vi "CAN_Command Standard.vi"(0 "Write":refnum<k21>, 1 "ID Response":string="18DAF255", 2 "Expression":string, 3 "CAN Command":string, 5 "Read":refnum<k21>, 9 "ID Request":string="18DA55F2", 11 "Numeric Request":u32 format="%x", 12 "Extended":bool=TRUE) -> (4 "Read out":refnum<k21>, 6 "Write out":refnum<k21>, 10 "ID String":string, 13 "Error Out":errorcluster, 14 "Timestamp":timestamp, 15 "Data String":string)   [LabVIEW 2023]
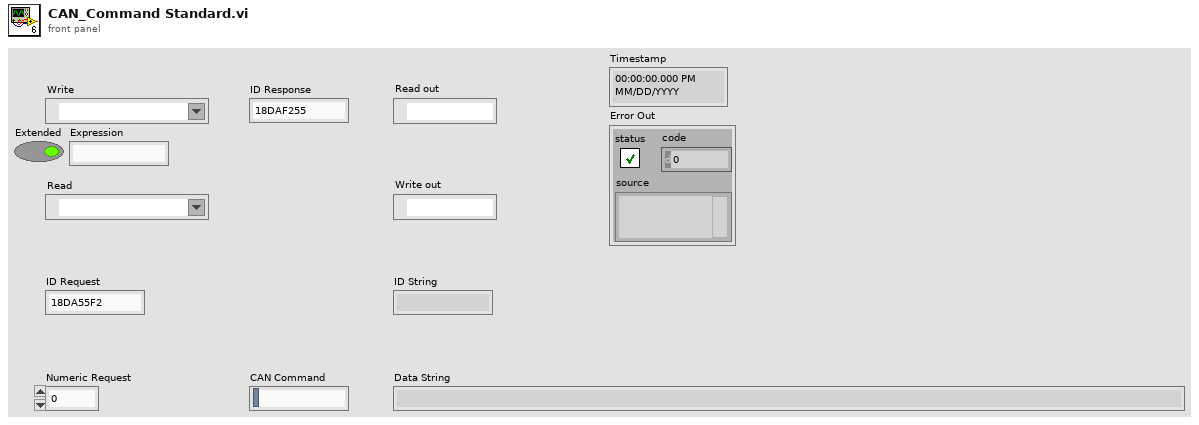
[diagram p1: front panel]
types:
  T1 = typedef "XNET Frame CAN.ctl" = cluster{"timestamp":timestamp, "payload":u8[], "identifier":u32, "type":T2, "extended?":bool, "echo?":bool}
  T2 = typedef "XNET Frame Type CAN.ctl" = u8
  T3 = cluster{"data[0]":T1, "data[1]":T1, "data[2]":T1, "data[3]":T1, "data[4]":T1, "data[5]":T1, "data[6]":T1, "data[7]":T1, "data[8]":T1}
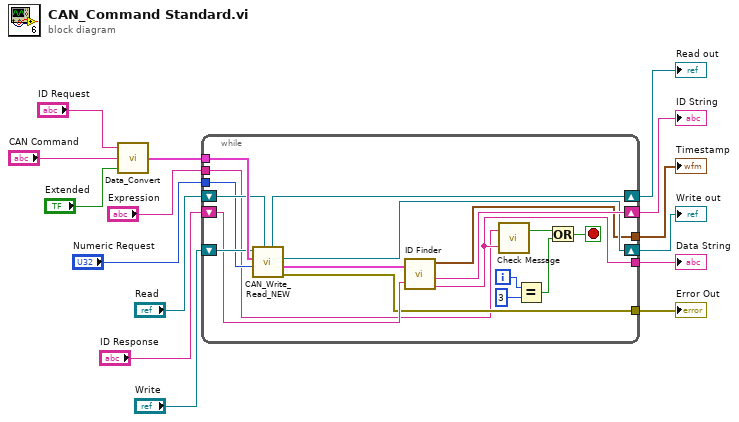
[diagram p0: block diagram]
diagram:
  n1 = call "Data_Convert.vi"("Extended"="Extended", "string"="CAN Command", "ID"="ID Request") -> ("CAN frame"=w13:T1)
  n2 = while {
    tunnel: [w17] -> w14
    tunnel: w13 -> [w31]
    tunnel: "Numeric Request" -> [w25]
    tunnel: [w24] -> w4
    tunnel: [w23] -> w2
    shift-right: [w27] -> w9
    shift-left: "Read" -> [w30]
    shift-right: [w28] -> w10
    shift-left: "Write" -> [w29]
    shift-right: [w33] -> w15
    shift-left: "ID Response" -> [w26]
    tunnel: "Expression" -> [w16]
    i -> [w22]
    stop <- w18 stop-if-true
    n3 = call "CAN_Write_Read_NEW.vi"("Read In"=w30, "Numeric Request"=w25, "CAN frame"=w31, "Write In"=w29) -> ("Error Out"=w23:errorcluster, "cluster"=w32:T3, "Write Out"=w28:refnum<k21>, "Read Out"=w27:refnum<k21>)  [unwired: 1 in, 1 out]
    n4 = call "ID Finder.vi"("cluster"=w32, "ID ESPERADO STRING"=w26) -> ("Timestamp"=w24:timestamp, "ID String"=w33:string, "Data String"=w17:string)  [unwired: 3 out]
    n5 = call "Check Message.vi"("Message"=w17, "Expression"=w16) -> ("Correct Message"=w20:bool)  [unwired: 1 in]
    n6 = Equal?(x=w22, y=3) -> (x = y?=w19:bool)
    n7 = Or(x=w20, y=w19) -> (x .or. y?=w18:bool)
  }
  "Data String" <- w14
  "ID String" <- w15
  "Write out" <- w10
  "Read out" <- w9
  "Timestamp" <- w4
  "Error Out" <- w2
